vi "F2.vi"(8 "s":dbl=1.0, 9 "d":dbl=10.0, 10 "w":dbl=10.0, 11 "a":dbl=1.0) -> (2 "F2":dbl format="%#_13g")   [LabVIEW 2021]
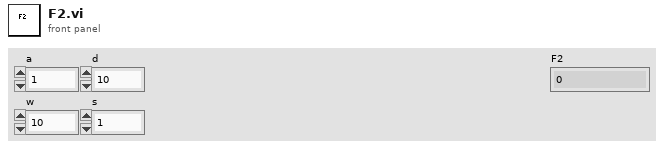
[diagram p1: front panel]
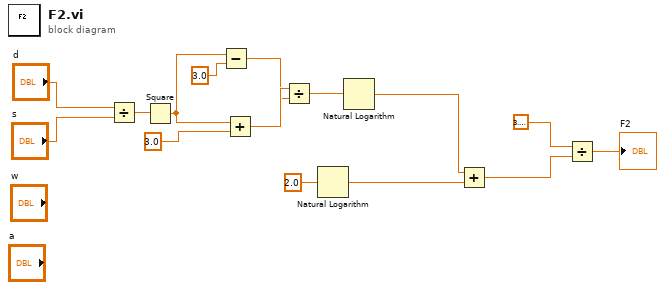
[diagram p0: block diagram]
diagram:
  n1 = Divide(x="d", y="s") -> (x/y=w10:dbl)
  n2 = Square(x=w10) -> (x^2=w8:dbl)
  n3 = Subtract(x=w8, y=3.0) -> (x-y=w5:dbl)
  n4 = Add(x=w8, y=3.0) -> (x+y=w6:dbl)
  n5 = Divide(x=w6, y=w5) -> (x/y=w4:dbl)
  n6 = Natural Logarithm(1:2.0) -> (0:w13:dbl)
  n7 = Natural Logarithm(1:w4) -> (0:w3:dbl)
  n8 = Add(x=w3, y=w13) -> (x+y=w2:dbl)
  n9 = Divide(x=3.141592653589793, y=w2) -> (x/y=→"F2":dbl)
